vi "MOD_RobotDriveMotors.vi"(6 "MotorIndex 2":T1=enum."Rear Right Motor", 7 "MotorIndex":T1, 8 "error in (no error)":errorcluster, 9 "RightSpeed":dbl, 10 "LeftSpeed":dbl, 11 "RobotDriveDevRef":T2={"DevStatus"={"status"=FALSE, "code"=0, "source"=""}, "Motors[]"=[], "Square Inputs"=FALSE, "Max Output"=1.0, "Isochronous"=FALSE}) -> (0 "error out":errorcluster, 3 "RobotDriveDevRef":T2={"DevStatus"={"status"=FALSE, "code"=0, "source"=""}, "Motors[]"=[], "Square Inputs"=FALSE, "Max Output"=1.0, "Isochronous"=FALSE})   [LabVIEW 2012]
doc: "Determines the motor configuration and sends the speed values to the appropriate motors.\n\nThis software is licensed. Open the labview\\readme\\WPI Robotics Library Open Source License.txt file for more information."
uses:
  <vilib>/Rock Robotics/WPI/RobotDrive/WPI_RobotDriveDevRef.ctl
  <vilib>/Rock Robotics/WPI/MotorControl/WPI_MotorControlDeviceRef.ctl
  <vilib>/Rock Robotics/SystemInterfaces/Typedef/FPGA_TypedefDigitalModule.ctl
  <vilib>/Rock Robotics/SystemInterfaces/DIO/FPGA_DIOPWMChannel.ctl
  <vilib>/Rock Robotics/WPI/PWM/WPI_PWMDeadband.ctl
  <vilib>/Rock Robotics/WPI/CAN/Jaguar/SubVIs/WPI_CANJaguar_ControlMode.ctl
  <vilib>/Rock Robotics/WPI/PWM/WPI_PWMTransform_ConPane.ctl
  <vilib>/Rock Robotics/WPI/RobotDrive/WPI_RobotDriveMotorSelectorEnum.ctl
  <vilib>/Rock Robotics/WPI/RobotDrive/WPI_RobotDriveSafetyCheck.vi
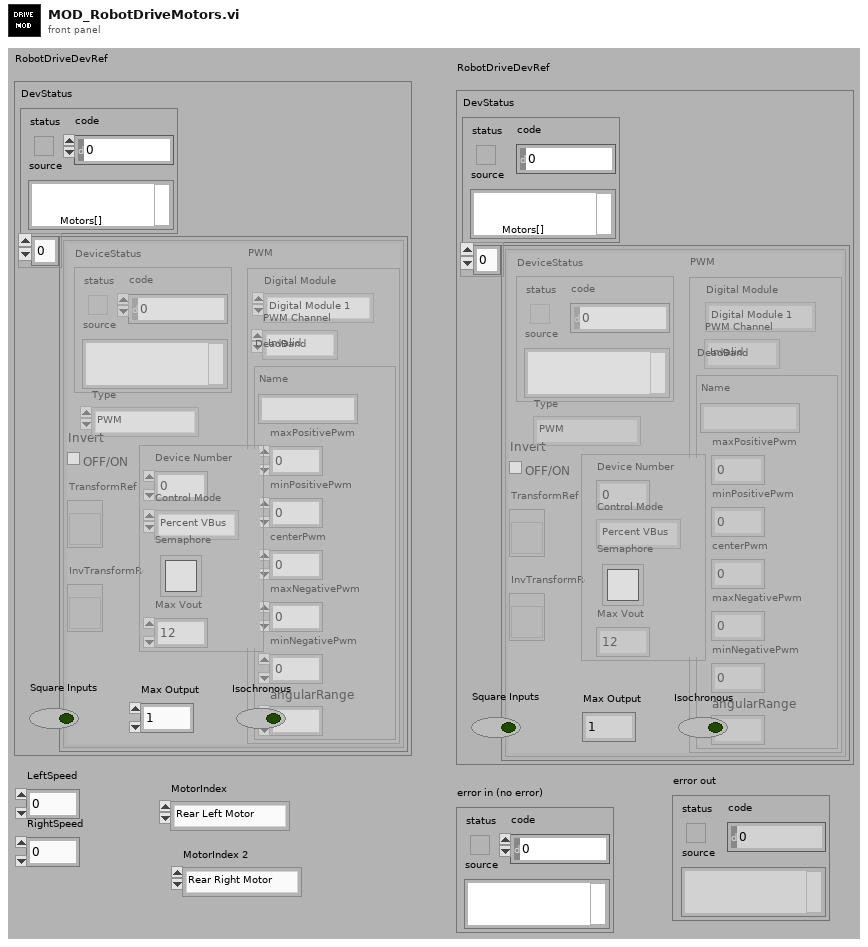
[diagram p1: front panel]
types:
  T1 = typedef "WPI_RobotDriveMotorSelectorEnum.ctl" = enum16{"Rear Left Motor", "Rear Right Motor", "Front Left Motor", "Front Right Motor"}
  T2 = typedef "WPI_RobotDriveDevRef.ctl" = cluster{"DevStatus":errorcluster, "Motors[]":T3[], "Square Inputs":bool, "Max Output":dbl, "Isochronous":bool}
  T3 = typedef "WPI_MotorControlDeviceRef.ctl" = cluster{"DeviceStatus":errorcluster, "Type":enum16{"PWM", "CAN"}, "PWM":cluster{"Digital Module":T4, "PWM Channel":T5, "DeadBand":T6}, "CAN":cluster{"Device Number":u8, "Control Mode":T7, "Semaphore":T8, "Max Vout":dbl}, "Invert":bool, "TransformRef":T9, "InvTransformRef":T9}
  T4 = typedef "FPGA_TypedefDigitalModule.ctl" = enum16{"Digital Module 1", "Digital Module 2"}
  T5 = typedef "FPGA_DIOPWMChannel.ctl" = enum8{"PWM 1", "PWM 2", "PWM 3", "PWM 4", "PWM 5", "PWM 6", "PWM 7", "PWM 8", "PWM 9", "PWM 10", "Invalid"}
  T6 = typedef "WPI_PWMDeadband.ctl" = cluster{"Name":string, "maxPositivePwm":i32, "minPositivePwm":i32, "centerPwm":i32, "maxNegativePwm":i32, "minNegativePwm":i32, "angularRange":u16}
  T7 = typedef "WPI_CANJaguar_ControlMode.ctl" = enum8{"Percent VBus", "Current", "Speed", "Position", "Voltage"}
  T8 = typedef "Semaphore RefNum" = refnum<k1>
  T9 = typedef "WPI_PWMTransform_ConPane.ctl" = refnum<vi>
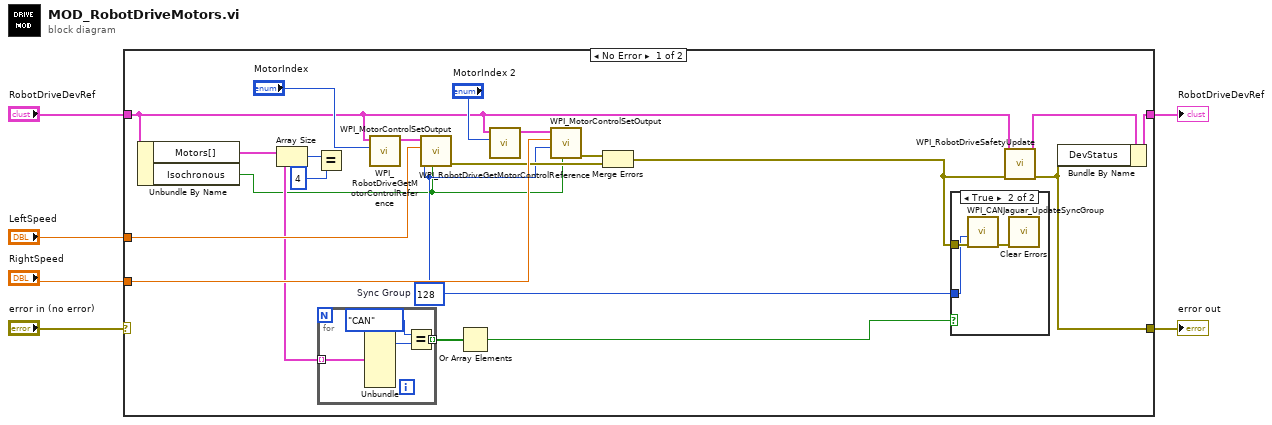
[diagram p0: block diagram]
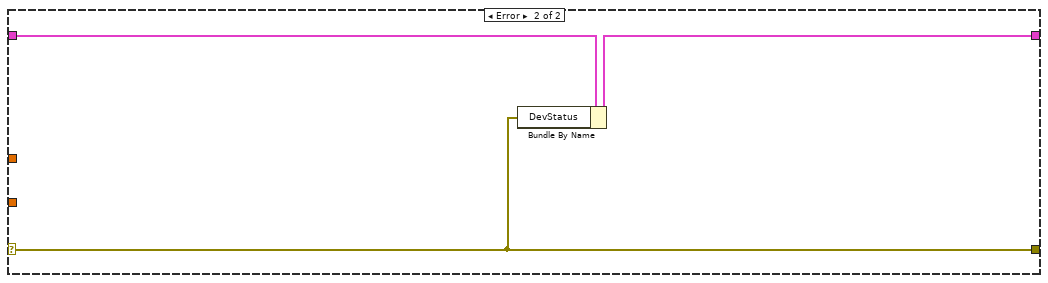
[diagram p3: hidden frame]
diagram:
  n1 = case shown="No Error" "error in (no error)" {
    selector: "error in (no error)" -> [_ w35]
    tunnel: "RobotDriveDevRef" -> [w20 w36]
    tunnel: [w17 w34] -> w5
    tunnel: "LeftSpeed" -> [w15 _]
    tunnel: "RightSpeed" -> [w16 _]
    tunnel: [w18 w35] -> w1
    frame No Error {
      w12 = u8 128  # Sync Group
      n2 = Unbundle By Name(w20) -> ("Motors[]"=w11:T3[], "Isochronous"=w8:bool)
      n3 = Array Size(array=w11) -> (size(s)=w26:i32)
      n4 = Equal?(x=w26, y=4) -> ()  [unwired: 1 out]
      n5 = for {
        tunnel: w11 -> [w30] mode=indexing
        tunnel: [w27] -> w10 mode=indexing
        n6 = Unbundle(w30) -> ("Type"=w29:enum16{"PWM", "CAN"})  [unwired: 6 out]
        n7 = Equal?(x=enum16{"PWM", "CAN"}."CAN" ("Type"), y=w29) -> (x = y?=w27:bool)
      }
      n8 = call <vilib>:"WPI_RobotDriveGetMotorControlReference.vi"("MotorIndex"="MotorIndex", "RobotDriveDevRef"=w20) -> ("MotorControlDeviceRef"=w23:T3)  [unwired: 9 out]
      n9 = call <vilib>:"WPI_MotorControlSetOutput.vi"("Isochronous"=w8, "Sync Group"=w12, "Output"=w15, "MotorControlDevRef"=w23) -> ("error out"=w13:errorcluster)  [unwired: 1 in, 6 out]
      n10 = Or Array Elements(Boolean array=w10) -> (logical OR=w9:bool)
      n11 = call <vilib>:"WPI_RobotDriveGetMotorControlReference.vi"("MotorIndex"="MotorIndex 2", "RobotDriveDevRef"=w20) -> ("MotorControlDeviceRef"=w24:T3)  [unwired: 9 out]
      n12 = call <vilib>:"WPI_MotorControlSetOutput.vi"("Isochronous"=w8, "Sync Group"=w12, "Output"=w16, "MotorControlDevRef"=w24) -> ("error out"=w14:errorcluster)  [unwired: 1 in, 6 out]
      n13 = Merge Errors(w14, w13) -> (w7:errorcluster)
      n14 = case shown="True" w9 {
        tunnel: w7 -> [_ w32]
        tunnel: w12 -> [_ w31]
        frame False {
        }
        frame True {
          n15 = call <vilib>:"WPI_CANJaguar_UpdateSyncGroup.vi"("error in (no error)"=w32, "Sync Group"=w31) -> ("error out"=w33:errorcluster)  [unwired: 9 out]
          n16 = call <vilib>:"Clear Errors.vi"("error in (no error)"=w33) -> ()  [unwired: 7 out]
        }
      }
      n17 = call <vilib>:"WPI_RobotDriveSafetyUpdate.vi"("error in (no error)"=w7, "RobotDriveDevRef"=w20) -> ("error out"=w18:errorcluster, "RobotDriveDevRef"=w19:T2)  [unwired: 8 out]
      n18 = Bundle By Name(cluster=w19, "DevStatus"=w18) -> (w17:T2)
    }
    frame Error {
      n19 = Bundle By Name(cluster=w36, "DevStatus"=w35) -> (w34:T2)
    }
  }
  "RobotDriveDevRef" <- w5
  "error out" <- w1
